vi "writeSGL.vi"(8 "error in (no error)":errorcluster, 10 "Input":sgl, 11 "M1M3SAL in":refnum<class "M1M3SAL.lvclass">) -> (0 "error out":errorcluster, 3 "M1M3SAL out":refnum<class "M1M3SAL.lvclass">)   [LabVIEW 2016, in "M1M3SupportCommunicator.lvlib" / "M1M3SAL.lvclass"]
uses:
  M1M3SAL.lvclass
  M1M3SAL.lvclass/M1M3SAL.ctl
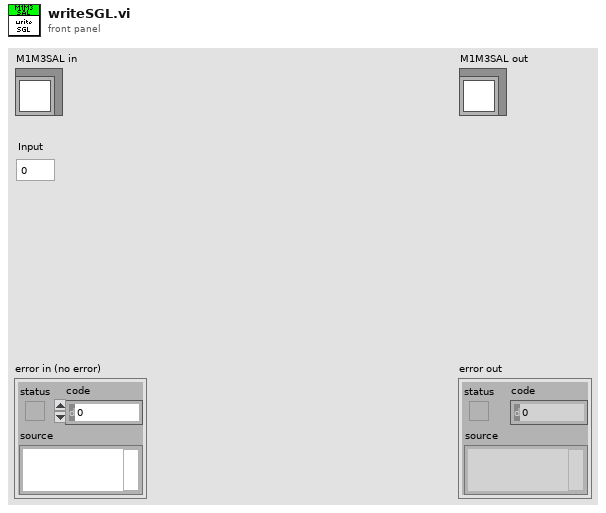
[diagram p1: front panel]
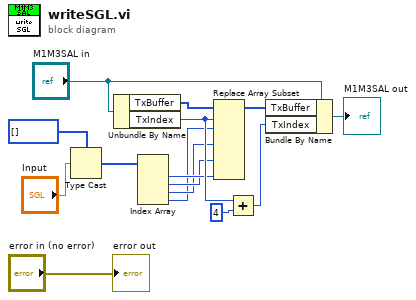
[diagram p0: block diagram]
diagram:
  n1 = Type Cast(type=u8[] [], x="Input") -> (*(type *) &x=w5:u8[])
  n2 = Unbundle By Name("M1M3SAL in") -> ("TxBuffer"=w13:u8[], "TxIndex"=w12:i32)
  n3 = Index Array(array=w5) -> (element #1=w4:u8, element #2=w3:u8, element #3=w2:u8, element #4=w1:u8)  [unwired: 4 in]
  n4 = Replace Array Subset(array=w13, new element #1=w1, index #1=w12, new element #2=w2, new element #3=w3, new element #4=w4) -> (w9:u8[])  [unwired: 3 in]
  n5 = Add(x=w12, y=4) -> (x+y=w10:i32)
  n6 = Bundle By Name(cluster="M1M3SAL in", "TxBuffer"=w9, "TxIndex"=w10) -> (→"M1M3SAL out":refnum<class "M1M3SAL.lvclass">)
  "error out" <- "error in (no error)"
